vi "FVI_GP2Y0A21YK0F_conversion.vi"(11 "Voltage":dbl) -> (3 "Numeric":dbl)   [LabVIEW 2018]
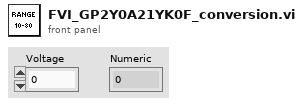
[diagram p1: front panel]
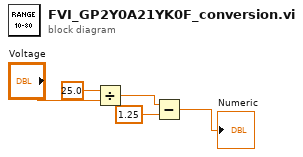
[diagram p0: block diagram]
diagram:
  n1 = Divide(x=25.0, y="Voltage") -> (x/y=w2:dbl)
  n2 = Subtract(x=w2, y=1.25) -> (x-y=→"Numeric":dbl)
